vi "setUp.vi"(8 "error in (no error)":errorcluster, 11 "reference in":refnum<class "testcase-csmhelper.lvclass">) -> (0 "error out":errorcluster, 3 "reference out":refnum<class "testcase-csmhelper.lvclass">)   [LabVIEW 2017, in "testcase-csmhelper.lvclass"]
doc: "setUp runs prior to the test method during test execution. Use this method to initialize any object data required by your tests."
uses:
  testcase-csmhelper.lvclass
  C:/Program Files (x86)/National Instruments/LabVIEW 2017/vi.lib/addons/_JKI Toolkits/VI Tester/TestCase.llb/TestCase.lvclass
  testcase-csmhelper.lvclass/testcase-csmhelper.ctl
  <vilib>/addons/_JKI Toolkits/VI Tester/TestCase.llb/TestCase.lvclass
  src/examples/NEVSTOP/Communicable State Machine(CSM)/1. Create a reuse Module/1. Create a reuse Module.lvlib
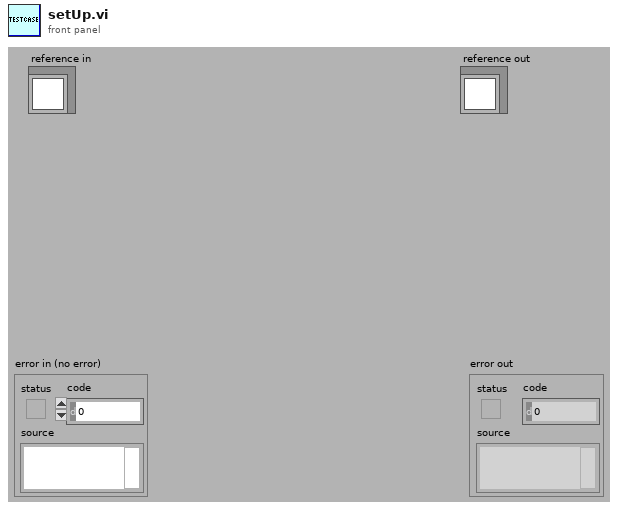
[diagram p1: front panel]
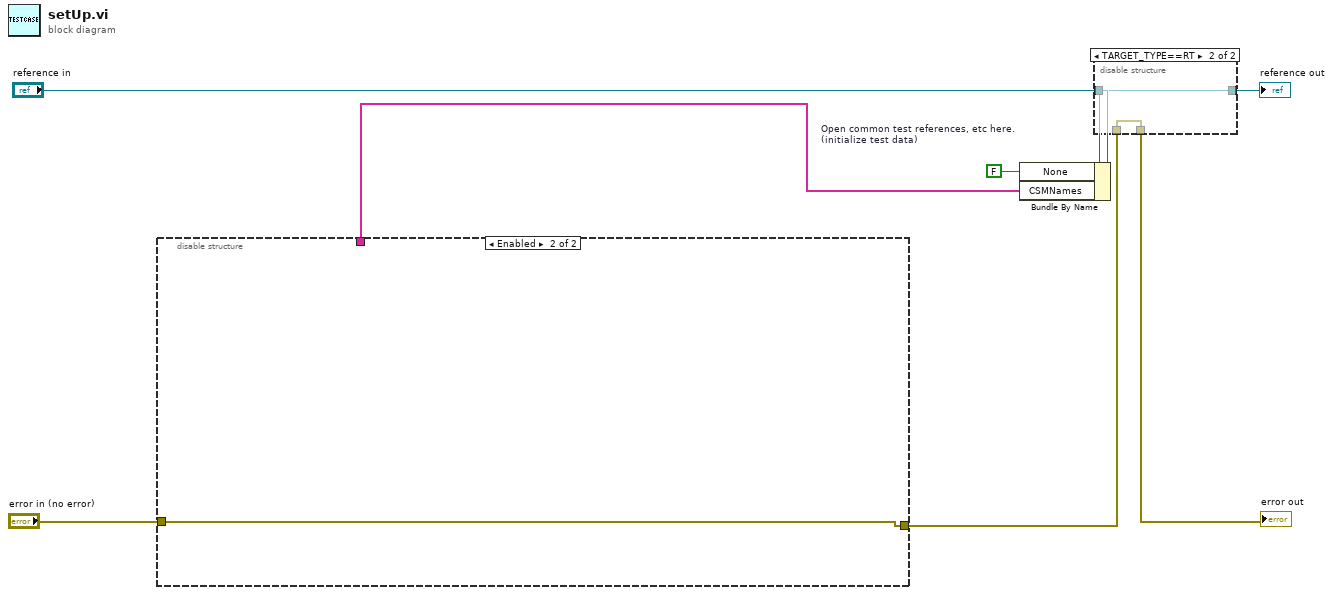
[diagram p0: block diagram]
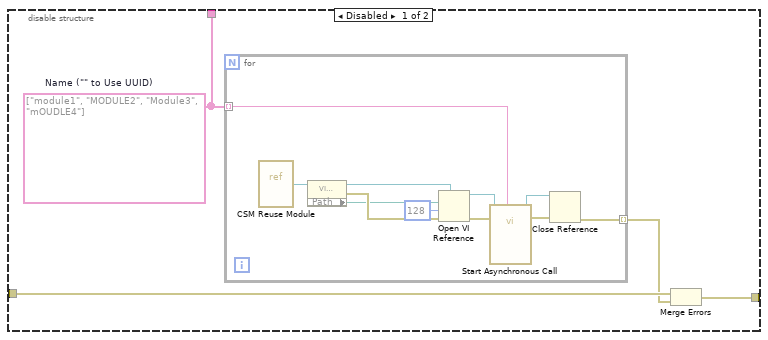
[diagram p2: hidden frame]
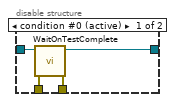
[diagram p3: hidden frame]
diagram:
  w3 = FALSE  # Open common test references, etc here. (initialize test data)
  n1 = disable-structure shown="Enabled" {
    disable-tunnel: "error in (no error)" -> [w12 w24]
    disable-tunnel: [w11 w24] -> w2
    disable-tunnel: [w9 _] -> w1
    frame Disabled {
      w9 = string[] ["module1", "MODULE2", "Module3", "mOUDLE4"]  # Name ("" to Use UUID)
      n2 = for {
        tunnel: w9 -> [w20] mode=indexing
        tunnel: [w13] -> w10 mode=indexing
        n3 = vi-ref "CSM Reuse Module.vi"() -> (w15:refnum<vi>)
        n4 = property class="VI (strict)"(reference=w15) -> (reference out=w19:refnum<vi>, error out=w17:errorcluster, "Path"=w16:path)  [unwired: 1 in]
        n5 = Open VI Reference(type specifier VI Refnum (for type only)=w19, vi path=w16, options=128, error in (no error)=w17) -> (vi reference=w18:refnum<vi>, error out=w14:errorcluster)  [unwired: 2 in]
        n6 = call-by-ref "Start Asynchronous Call"(reference=w18, error in=w14, "Name(\"\" to use uuid)"=w20) -> (reference out=w22:refnum<vi>, error out=w21:errorcluster)  [unwired: 11 in]
        n7 = Close Reference(reference=w22, error in (no error)=w21) -> (error out=w13:errorcluster)
      }
      n8 = Merge Errors(w12, w10) -> (w11:errorcluster)
    }
    frame Enabled {
    }
  }
  n9 = Bundle By Name(cluster="reference in", "None"=w3, "CSMNames"=w1) -> (w4:refnum<class "testcase-csmhelper.lvclass">)
  n10 = disable-structure shown="TARGET_TYPE==RT" {
    disable-tunnel: w2 -> [w28 w29]
    disable-tunnel: [w27 w29] -> w7
    disable-tunnel: [w26 w30] -> w5
    disable-tunnel: w4 -> [w25 w30]
    frame condition #0 (active) {
      n11 = call <vilib>:"WaitOnTestComplete.vi"("error in (no error)"=w28, "TestCase in"=w25) -> ("error out"=w27:errorcluster, "TestCase out"=w26:refnum<class "testcase-csmhelper.lvclass">)  [unwired: 8 in]
    }
    frame condition #1 {
    }
  }
  "error out" <- w7
  "reference out" <- w5
